vi "IFNoise-Init Hardware.vi"(0 "AO Buffer":dbl[](array[numeric]), 1 "Speaker":T1, 5 "Sampling rate (Hz)":dbl, 7 "Npts":i32, 9 "Attenuation (dB)":dbl, 11 "error in (no error)":errorcluster, 12 "Input source":enum16{"Probe Mic", "Cal Mic", "Voltage Only"}(ring)) -> (8 "AO Channels":i32[](array[numeric]), 15 "error out":errorcluster)   [LabVIEW 2015]
uses:
  Misc VIs/Connection Manager/Type Defs/Input sources.ctl
  Misc VIs/Connection Manager/Type Defs/Output sources.ctl
  PXI DAQ VIs/DAQ Engine VIs/AO Gain and Multiplier VIs/PXI Multipliers to AO Gains (1D).vi
  Utility VIs/Type Defs/Speaker ring.ctl
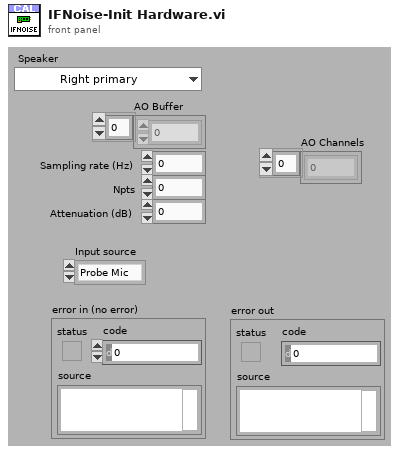
[diagram p1: front panel]
types:
  T1 = typedef "Speaker ring.ctl" = enum16{"Right primary", "Right secondary", "Left primary", "Left secondary"}
  T2 = typedef "Output sources.ctl" = u16
  T3 = typedef "Input sources.ctl" = u16
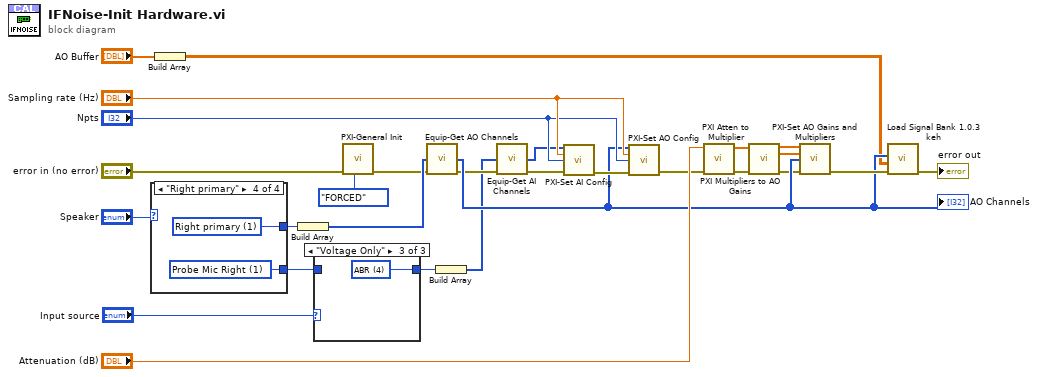
[diagram p0: block diagram]
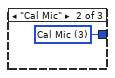
[diagram p3: hidden frame]
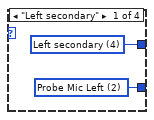
[diagram p4: hidden frame]
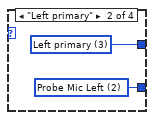
[diagram p5: hidden frame]
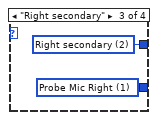
[diagram p6: hidden frame]
diagram:
  n1 = case shown="\"Right primary\"" "Speaker" {
    tunnel: [w30 w32 w34 w36] -> w8
    tunnel: [w29 w31 w33 w35] -> w2
    frame "Left secondary" {
      w30 = T2 4 items=["--unused--", "Right primary", "Right secondary", "Left primary", "Left secondary", "Shocks", "Startle", "Background"] ("Ring")
      w29 = T3 2 items=["--unused--", "Probe Mic Right", "Probe Mic Left", "Cal Mic", "ABR", "CAP Right", "CAP Left", "Startle piezo", "Temperature", "Heart rate"] ("Ring")
    }
    frame "Left primary" {
      w32 = T2 3 items=["--unused--", "Right primary", "Right secondary", "Left primary", "Left secondary", "Shocks", "Startle", "Background"] ("Ring")
      w31 = T3 2 items=["--unused--", "Probe Mic Right", "Probe Mic Left", "Cal Mic", "ABR", "CAP Right", "CAP Left", "Startle piezo", "Temperature", "Heart rate"] ("Ring")
    }
    frame "Right secondary" {
      w34 = T2 2 items=["--unused--", "Right primary", "Right secondary", "Left primary", "Left secondary", "Shocks", "Startle", "Background"] ("Ring")
      w33 = T3 1 items=["--unused--", "Probe Mic Right", "Probe Mic Left", "Cal Mic", "ABR", "CAP Right", "CAP Left", "Startle piezo", "Temperature", "Heart rate"] ("Ring")
    }
    frame "Right primary" {
      w36 = T2 1 items=["--unused--", "Right primary", "Right secondary", "Left primary", "Left secondary", "Shocks", "Startle", "Background"] ("Ring")
      w35 = T3 1 items=["--unused--", "Probe Mic Right", "Probe Mic Left", "Cal Mic", "ABR", "CAP Right", "CAP Left", "Startle piezo", "Temperature", "Heart rate"] ("Ring")
    }
  }
  n2 = Build Array("AO Buffer") -> (w7:dbl[][])
  n3 = Build Array(w8) -> (w12:T2[])
  n4 = case shown="\"Voltage Only\"" "Input source" {
    tunnel: w2 -> [w37 _ _]
    tunnel: [w37 w38 w39] -> w1
    frame "Probe Mic", Default {
    }
    frame "Cal Mic" {
      w38 = T3 3 items=["--unused--", "Probe Mic Right", "Probe Mic Left", "Cal Mic", "ABR", "CAP Right", "CAP Left", "Startle piezo", "Temperature", "Heart rate"] ("Ring")
    }
    frame "Voltage Only" {
      w39 = T3 4 items=["--unused--", "Probe Mic Right", "Probe Mic Left", "Cal Mic", "ABR", "CAP Right", "CAP Left", "Startle piezo", "Temperature", "Heart rate"] ("Ring")
    }
  }
  n5 = call "PXI-General Init.vi"("Double Buffer Mode"=enum32{"OFF", "ENABLED", "FORCED"}."FORCED", "error in (no error)"="error in (no error)") -> ("error out"=w5:errorcluster)  [unwired: 9 in]
  n6 = call "Equip-Get AO Channels.vi"("Outputs"=w12, "error in (no error)"=w5) -> ("AO Channels"=w19:i32[], "error out"=w14:errorcluster)  [unwired: 12 in]
  "AO Channels" <- w19
  n7 = Build Array(w1) -> (w13:T3[])
  n8 = call "Equip-Get AI Channels.vi"("Inputs"=w13, "error in (no error)"=w14) -> ("AI Channels"=w21:i32[], "error out"=w6:errorcluster)  [unwired: 12 in]
  n9 = call "PXI-Set AI Config.vi"("AI Channels"=w21, "Sampling Rate (Hz)"="Sampling rate (Hz)", "Buffer Size"="Npts", "error in (no error)"=w6) -> ("error out"=w20:errorcluster)  [unwired: 11 in]
  n10 = call "PXI-Set AO Config.vi"("AO Channels"=w19, "Sampling Rate (Hz)"="Sampling rate (Hz)", "Buffer Size"="Npts", "error in (no error)"=w20) -> ("error out"=w18:errorcluster)  [unwired: 11 in]
  n11 = call "PXI Atten to Multiplier.vi"("error in (no error)"=w18, "Attenuation"="Attenuation (dB)") -> ("error out"=w9:errorcluster, "Multiplier setting"=w10:dbl[])  [unwired: 8 in]
  n12 = call-poly "PXI Multipliers to AO Gains.vi"("Multipliers in"=w10, "error in (no error)"=w9) -> ("Multipliers out"=w16:dbl[], "Gains"=w17:dbl[], "error out"=w15:errorcluster)  [unwired: 11 in]
  n13 = call "PXI-Set AO Gains and Multipliers.vi"("Multipliers"=w16, "Gains"=w17, "AO Channels"=w19, "error in (no error)"=w15) -> ("error out"=w23:errorcluster)  [unwired: 11 in]
  n14 = call "Load Signal Bank 1.0.3 keh.vi"("error in (no error)"=w23, "Input array"=w7, "Active AO Array"=w19) -> ("error out"=→"error out":errorcluster)  [unwired: 3 in, 1 out]
